vi "Build_Asylum_ReadGroup.vi"(8 "error in (no error)":errorcluster, 10 "wave":string, 11 "groupName":string) -> (0 "error out":errorcluster, 3 "Command":string)   [LabVIEW 2019]
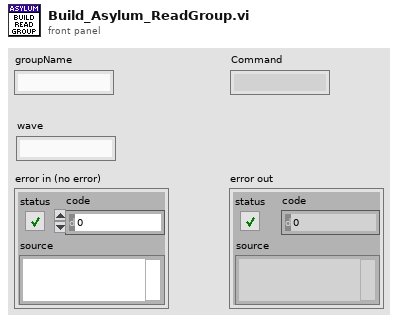
[diagram p1: front panel]
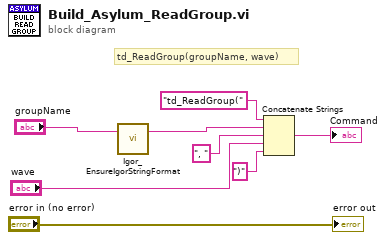
[diagram p0: block diagram]
diagram:
  # "td_ReadGroup(groupName, wave)"
  n1 = call <userlib>:"Igor_EnsureIgorStringFormat.vi"("Value"="groupName") -> ("Value"=w7:string)  [unwired: 2 in]
  n2 = Concatenate Strings("td_ReadGroup(" ("string"), w7, ", " ("string"), "wave", ")" ("string")) -> (→"Command":string)
  "error out" <- "error in (no error)"
